vi "Two interface Max.vi"(9 "Width":u32, 11 "S":dbl[](array[numeric])) -> (2 "MAX_Index":i32, 3 "INDEX":i32[](array[numeric]))   [LabVIEW 2015, in "Boimetry Processing.lvlib"]
uses:
  Boimetry Processing.lvlib
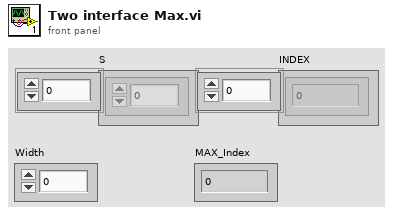
[diagram p1: front panel]
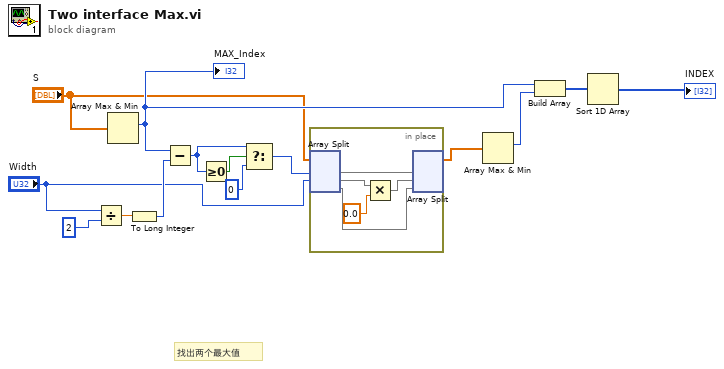
[diagram p0: block diagram]
diagram:
  # "找出两个最大值"
  n1 = Divide(x="Width", y=u32 2) -> (x/y=w13:dbl)
  n2 = Array Max & Min(array="S") -> (max index (indices)=w5:i32)  [unwired: 3 out]
  "MAX_Index" <- w5
  n3 = To Long Integer(number=w13) -> (32bit integer=w12:i32)
  n4 = Subtract(x=w5, y=w12) -> (x-y=w9:i32)
  n5 = Greater Or Equal To 0?(x=w9) -> (x >= 0?=w10:bool)
  n6 = Select(t=w9, s=w10, f=u32 0) -> (s? t:f=w3:u32)
  n7 = in-place {
    n8 = in-place-split #1("S", w3, "Width") -> (w19:dbl[], w17:dbl[], w15:dbl[])
    n9 = Multiply(x=w17, y=0.0) -> (x*y=w18:dbl[])
    n10 = in-place-split #1(w19, w18, w15) -> (w1:dbl[])  [unwired: 2 out]
  }
  n11 = Array Max & Min(array=w1) -> (max index (indices)=w11:i32)  [unwired: 3 out]
  n12 = Build Array(w5, w11) -> (w6:i32[])
  n13 = Sort 1D Array(array=w6) -> (sorted array=→"INDEX":i32[])
